vi "Create Message VI (from Template).vi"(7 "replace string in template":string="package_templatemessage", 8 "error in (no error)":errorcluster, 9 "template VI name":string="Get package_templatemessage.vi", 10 "RPC Message Name":string, 11 "RPC Messages Folder (ProjectItem) in":refnum<vi>) -> (0 "error out":errorcluster, 1 "Created?":bool, 2 "Getter VI out":refnum<vi>, 3 "RPC Messages Folder (ProjectItem) out":refnum<vi>)   [LabVIEW 2019, in "gRPC Template Creation Utility.lvlib"]
uses:
  gRPC Template Creation Utility.lvlib
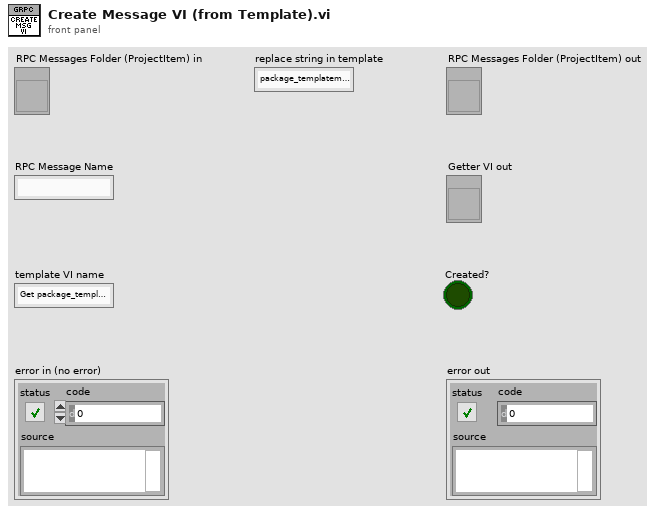
[diagram p1: front panel]
types:
  T1 = enum32{"invalid VI type", "Standard VI", "Control VI", "Global VI", "Polymorphic VI", "Configuration VI", "SubSystem", "Facade VI", "Method VI"}
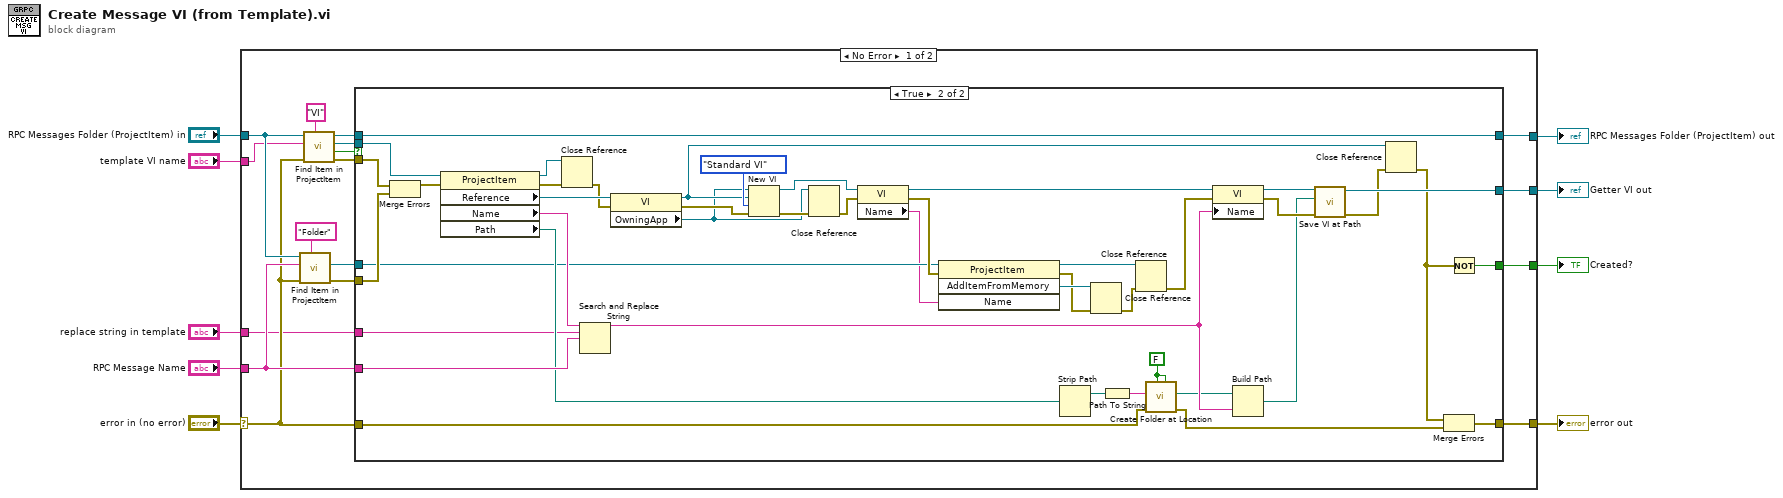
[diagram p0: block diagram]
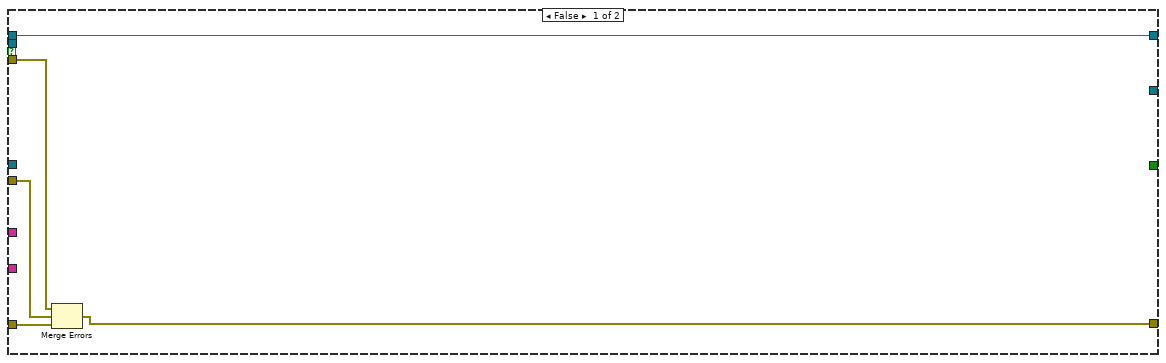
[diagram p2: hidden frame]
diagram:
  n1 = case shown="No Error" "error in (no error)" {
    selector: "error in (no error)" -> [w16 w76]
    tunnel: "RPC Message Name" -> [w26 _]
    tunnel: "RPC Messages Folder (ProjectItem) in" -> [w25 w77]
    tunnel: [w24 w76] -> w7
    tunnel: [w13 w77] -> w6
    tunnel: [w21 _] -> w5
    tunnel: [w12 _] -> w3
    tunnel: "template VI name" -> [w11 _]
    tunnel: "replace string in template" -> [w10 _]
    frame No Error {
      n2 = call "Find Item in ProjectItem.vi"("Item Type"="Folder", "error in (no error)"=w16, "Name"=w26, "ProjectItem in"=w25) -> ("error out"=w23:errorcluster, "Item Refnum out"=w20:refnum<vi>)  [unwired: 4 in, 2 out]
      n3 = call "Find Item in ProjectItem.vi"("Item Type"="VI", "error in (no error)"=w16, "Name"=w11, "ProjectItem in"=w25) -> ("error out"=w22:errorcluster, "Found ?"=w15:bool, "Item Refnum out"=w19:refnum<vi>, "ProjectItem out"=w14:refnum<vi>)  [unwired: 4 in]
      n4 = case shown="True" w15 {
        tunnel: w26 -> [_ w75]
        tunnel: [w29 w72] -> w24
        tunnel: w23 -> [w27 w70]
        tunnel: w22 -> [w28 w68]
        tunnel: [_ w66] -> w21
        tunnel: w20 -> [_ w55]
        tunnel: w19 -> [_ w51]
        tunnel: w16 -> [w30 w50]
        tunnel: w14 -> [w31 w49]
        tunnel: [w31 w49] -> w13
        tunnel: [_ w46] -> w12
        tunnel: w10 -> [_ w39]
        frame False {
          n5 = Merge Errors(w28, w27, w30) -> (w29:errorcluster)
        }
        frame True {
          w67 = FALSE ("Use Relative (F)")
          n6 = Merge Errors(w68, w70) -> (w69:errorcluster)
          n7 = property class="ProjectItem"(reference=w51, error in=w69) -> (reference out=w74:refnum<vi>, error out=w73:errorcluster, "Reference"=w38:refnum<vi>, "Name"=w58:string, "Path"=w57:path)
          n8 = Close Reference(reference=w74, error in (no error)=w73) -> (error out=w36:errorcluster)
          n9 = Search and Replace String(input string=w58, search string=w39, replace string=w75) -> (result string=w62:string)  [unwired: 5 in, 3 out]
          n10 = property class="VI"(reference=w38, error in=w36) -> (reference out=w37:refnum<vi>, error out=w35:errorcluster, "OwningApp"=w32:refnum<vi>)
          n11 = New VI(8:w35, 9:T1."Standard VI" ("vi type (standard vi)"), 10:w37, 11:w32) -> (0:w34:errorcluster, 3:w52:refnum<vi>)  [unwired: 3 out]
          n12 = Close Reference(reference=w32, error in (no error)=w34) -> (error out=w33:errorcluster)
          n13 = property class="VI"(reference=w52, error in=w33) -> (reference out=w59:refnum<vi>, error out=w60:errorcluster, "Name"=w54:string)
          n14 = invoke class="ProjectItem" method="AddItemFromMemory"(reference=w55, error in=w60, "Name"=w54) -> (reference out=w48:refnum<vi>, error out=w44:errorcluster, "AddItemFromMemory"=w45:refnum<vi>)  [unwired: 1 in, 1 out]
          n15 = Strip Path(path=w57) -> (stripped path=w40:path)  [unwired: 1 out]
          n16 = Close Reference(reference=w45, error in (no error)=w44) -> (error out=w43:errorcluster)
          n17 = Path To String(path=w40) -> (string=w56:string)
          n18 = Close Reference(reference=w48, error in (no error)=w43) -> (error out=w47:errorcluster)
          n19 = call "Create Folder at Location.vi"("Override existing (F)"=w67, "Use Relative (F)"=w67, "Error In"=w50, "Path"=w56) -> ("Error Out"=w71:errorcluster, "Full path out"=w61:path)  [unwired: 5 in, 1 out]
          n20 = property class="VI"(reference=w59, error in=w47, "Name"=w62) -> (reference out=w63:refnum<vi>, error out=w65:errorcluster)
          n21 = Build Path(base path=w61, name or relative path=w62) -> (appended path=w64:path)
          n22 = call "Save VI at Path.vi"("error in (no error)"=w65, "Path"=w64, "VI in"=w63) -> ("error out"=w42:errorcluster, "VI out"=w66:refnum<vi>)  [unwired: 6 in, 1 out]
          n23 = Close Reference(reference=w37, error in (no error)=w42) -> (error out=w41:errorcluster)
          n24 = Merge Errors(w41, w71) -> (w72:errorcluster)
          n25 = Not(x=w41) -> (.not. x?=w46:bool)
        }
      }
    }
    frame Error {
    }
  }
  "error out" <- w7
  "RPC Messages Folder (ProjectItem) out" <- w6
  "Getter VI out" <- w5
  "Created?" <- w3
